vi "Register Private ADS Symbol Version Change Event Callbacks.vi"(8 "error in (no error)":errorcluster, 11 "TwinCAT ADS in":refnum<class "TwinCAT ADS.lvclass">) -> (0 "error out":errorcluster, 3 "TwinCAT ADS out":refnum<class "TwinCAT ADS.lvclass">)   [LabVIEW 2018, in "TwinCAT ADS.lvclass"]
uses:
  TwinCAT ADS.lvclass
  TwinCAT ADS.lvclass/TwinCAT ADS.ctl
  TwinCAT.Ads
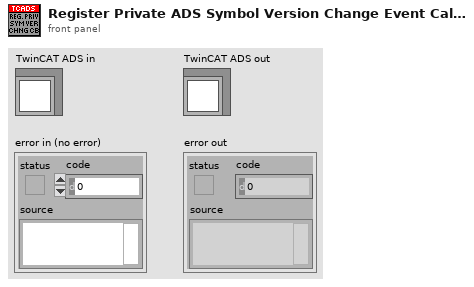
[diagram p1: front panel]
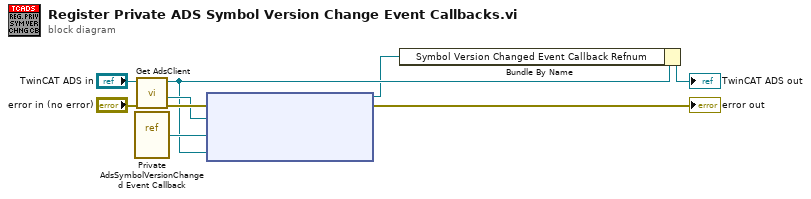
[diagram p0: block diagram]
diagram:
  n1 = vi-ref "Private AdsSymbolVersionChanged Event Callback.vi"() -> ("vi reference"=w6:refnum<vi>)
  n2 = call "Get AdsClient.vi"("error in (no error)"="error in (no error)", "TwinCAT ADS in"="TwinCAT ADS in") -> ("error out"=w9:errorcluster, ".NET TcAdsClient"=w5:refnum<k24>, "TwinCAT ADS out"=w4:refnum<class "TwinCAT ADS.lvclass">)  [unwired: 7 in]
  n3 = node(w9, w5, w6, w4) -> (w3:refnum<k27>, →"error out":errorcluster)  [unwired: 1 in]
  n4 = Bundle By Name(cluster=w4, "Symbol Version Changed Event Callback Refnum"=w3) -> (→"TwinCAT ADS out":refnum<class "TwinCAT ADS.lvclass">)
